vi "MGCC_StaEst_main_v2.vi"() -> ()   [LabVIEW 2016]
uses:
  <vilib>/imath/engines/lvmath2/RunTimeEngine/IndexRead/NIMS M(S,S).vi
  <instcachedir>/0/NIMS M(S,S)_AC51E74150A542F7991B9634C66F3096.lvgen/NIMS M(S,S)_AC51E74150A542F7991B9634C66F3096_001.vi
  <vilib>/imath/engines/lvmath2/RunTimeEngine/BuiltInFunctions/abs/NIMS_abs(signed).vi
  <instcachedir>/0/NIMS_abs(signed)_C4FCB8E6058B49B797C7C8D53CA5F6EC.lvgen/NIMS_abs(signed)_C4FCB8E6058B49B797C7C8D53CA5F6EC_002.vi
  <vilib>/imath/engines/lvmath2/RunTimeEngine/RunTimeType/NIMS_RunTimeType_From StrictType (excl LVString).vi
  <instcachedir>/0/NIMS_RunTimeType_From StrictType (excl LVString)_BBF44FB49F834B71AF7A14CCEDF8BECD.lvgen/NIMS_RunTimeType_From StrictType (excl LVString)_BBF44FB49F834B71AF7A14CCEDF8BECD_031.vi
  <vilib>/imath/engines/lvmath2/RunTimeEngine/Struct/NIMS_StructSetField.vi
  <vilib>/imathl/engines/lvmath/Functions/Error Handling/Create Error.vi
  <vilib>/imath/engines/lvmath2/RunTimeEngine/Struct/NIMS_StructGetField.vi
  <vilib>/imath/engines/lvmath2/RunTimeEngine/RunTimeType/NIMS_RunTimeType_To Numeric.vi
  <instcachedir>/0/NIMS_RunTimeType_To Numeric_19D51BCABB82435A94073491761E42EE.lvgen/NIMS_RunTimeType_To Numeric_19D51BCABB82435A94073491761E42EE_008.vi
  <instcachedir>/0/NIMS_RunTimeType_From StrictType (excl LVString)_BBF44FB49F834B71AF7A14CCEDF8BECD.lvgen/NIMS_RunTimeType_From StrictType (excl LVString)_BBF44FB49F834B71AF7A14CCEDF8BECD_000.vi
  <instcachedir>/0/NIMS_RunTimeType_To Numeric_19D51BCABB82435A94073491761E42EE.lvgen/NIMS_RunTimeType_To Numeric_19D51BCABB82435A94073491761E42EE_000.vi
  <vilib>/imath/engines/lvmath2/RunTimeEngine/IndexRead/NIMS M($,R2).vi
  <instcachedir>/0/NIMS M($,R2)_D9380E19261A4ADFB2D364AF6959C6EF.lvgen/NIMS M($,R2)_D9380E19261A4ADFB2D364AF6959C6EF_000.vi
  <instcachedir>/0/NIMS_RunTimeType_From StrictType (excl LVString)_BBF44FB49F834B71AF7A14CCEDF8BECD.lvgen/NIMS_RunTimeType_From StrictType (excl LVString)_BBF44FB49F834B71AF7A14CCEDF8BECD_009.vi
  <vilib>/imath/engines/lvmath2/RunTimeEngine/BuiltInFunctions/imag/NIMS_imag(Complex).vi
  <instcachedir>/0/NIMS_imag(Complex)_3180D40D00C843A49C2B33397F857BF3.lvgen/NIMS_imag(Complex)_3180D40D00C843A49C2B33397F857BF3_001.vi
  <instcachedir>/0/NIMS_abs(signed)_C4FCB8E6058B49B797C7C8D53CA5F6EC.lvgen/NIMS_abs(signed)_C4FCB8E6058B49B797C7C8D53CA5F6EC_003.vi
  <vilib>/imath/engines/lvmath2/RunTimeEngine/BuiltInFunctions/angle/NIMS_angle.vi
  <instcachedir>/0/NIMS_angle_6DDAE2BD99E0421EB990B6436E94D88F.lvgen/NIMS_angle_6DDAE2BD99E0421EB990B6436E94D88F_001.vi
  <instcachedir>/0/NIMS_RunTimeType_To Numeric_19D51BCABB82435A94073491761E42EE.lvgen/NIMS_RunTimeType_To Numeric_19D51BCABB82435A94073491761E42EE_003.vi
  <instcachedir>/0/NIMS_abs(signed)_C4FCB8E6058B49B797C7C8D53CA5F6EC.lvgen/NIMS_abs(signed)_C4FCB8E6058B49B797C7C8D53CA5F6EC_005.vi
  <vilib>/imath/engines/lvmath2/RunTimeEngine/VariableToken/Support/NIMS_Matrix Boolean Index to I32 Index.vi
  <vilib>/imath/engines/lvmath2/RunTimeEngine/IndexReplace/NIMS M(V)=S.vi
  <instcachedir>/0/NIMS M(V)=S_F2304187E1344F60ABCBE5C5CC0920F9.lvgen/NIMS M(V)=S_F2304187E1344F60ABCBE5C5CC0920F9_000.vi
  <instcachedir>/0/NIMS M($,R2)_D9380E19261A4ADFB2D364AF6959C6EF.lvgen/NIMS M($,R2)_D9380E19261A4ADFB2D364AF6959C6EF_001.vi
  <instcachedir>/0/NIMS_RunTimeType_From StrictType (excl LVString)_BBF44FB49F834B71AF7A14CCEDF8BECD.lvgen/NIMS_RunTimeType_From StrictType (excl LVString)_BBF44FB49F834B71AF7A14CCEDF8BECD_032.vi
  <instcachedir>/0/NIMS_RunTimeType_From StrictType (excl LVString)_BBF44FB49F834B71AF7A14CCEDF8BECD.lvgen/NIMS_RunTimeType_From StrictType (excl LVString)_BBF44FB49F834B71AF7A14CCEDF8BECD_024.vi
  LabVIEW Data/MathScriptVIs/MCStatic_36913154532_e94463401f82ecd62a182994faf25da2.vi
  <instcachedir>/0/MCStatic_36913154532_e94463401f82ecd62a182994faf25da2_D5C5374974BB412B8DCFE71036B3BD4D.lvgen/MCStatic_36913154532_e94463401f82ecd62a182994faf25da2_D5C5374974BB412B8DCFE71036B3BD4D_000.vi
  <instcachedir>/0/NIMS_RunTimeType_To Numeric_19D51BCABB82435A94073491761E42EE.lvgen/NIMS_RunTimeType_To Numeric_19D51BCABB82435A94073491761E42EE_009.vi
  <instcachedir>/0/NIMS_RunTimeType_To Numeric_19D51BCABB82435A94073491761E42EE.lvgen/NIMS_RunTimeType_To Numeric_19D51BCABB82435A94073491761E42EE_010.vi
  <vilib>/imath/engines/lvmath2/RunTimeEngine/BuiltInFunctions/size/NIMS_I32=size(GCol,I32).vi
  <instcachedir>/0/NIMS_I32=size(GCol,I32)_3BEAC9C04C22472CB193ADA08E7FE41C.lvgen/NIMS_I32=size(GCol,I32)_3BEAC9C04C22472CB193ADA08E7FE41C_000.vi
  <vilib>/imath/engines/lvmath2/RunTimeEngine/RangeToken/NIMS_Range_R2 - Integer.vi
  <instcachedir>/0/NIMS_Range_R2 - Integer_89B873E74E6E489885E44F751DD9C6BF.lvgen/NIMS_Range_R2 - Integer_89B873E74E6E489885E44F751DD9C6BF_000.vi
  <vilib>/imath/engines/lvmath2/RunTimeEngine/CommandStatement/MC_CommandStatement_break.vi
  <vilib>/imath/engines/lvmath2/RunTimeEngine/IndexRead/NIMS V(S).vi
  <instcachedir>/0/NIMS V(S)_0488751826AF41519A22953C041130DC.lvgen/NIMS V(S)_0488751826AF41519A22953C041130DC_002.vi
  <vilib>/imath/engines/lvmath2/RunTimeEngine/MatrixToken/NIMS_MatrixToken_M_RV.vi
  <instcachedir>/0/NIMS_MatrixToken_M_RV_EE14907D4B194E829889005D2F556E9C.lvgen/NIMS_MatrixToken_M_RV_EE14907D4B194E829889005D2F556E9C_002.vi
  <vilib>/imath/engines/lvmath2/RunTimeEngine/ErrorHandling/NIMS_Create Error From Enums.vi
  LabVIEW Data/MathScriptVIs/MCStatic_36913154532_cdc492c47a81eb15c08497af6b311993.vi
  <instcachedir>/0/MCStatic_36913154532_cdc492c47a81eb15c08497af6b311993_54503743F61444378DD671EE6F584E70.lvgen/MCStatic_36913154532_cdc492c47a81eb15c08497af6b311993_54503743F61444378DD671EE6F584E70_000.vi
  <vilib>/imath/engines/lvmath2/RunTimeEngine/RangeToken/NIMS_Range.vi
  <instcachedir>/0/NIMS_Range_A7C094595B484CA7AF10685B02D808ED.lvgen/NIMS_Range_A7C094595B484CA7AF10685B02D808ED_000.vi
  <vilib>/imath/engines/lvmath2/RunTimeEngine/MatrixToken/NIMS_MatrixToken_M_SorCV.vi
  <instcachedir>/0/NIMS_MatrixToken_M_SorCV_D3266533510A4291A747E91CF193467A.lvgen/NIMS_MatrixToken_M_SorCV_D3266533510A4291A747E91CF193467A_000.vi
  LabVIEW Data/MathScriptVIs/MCStatic_36913154532_c8cdcb96f1d039e13ab6944736b2cbcd.vi
  <instcachedir>/0/MCStatic_36913154532_c8cdcb96f1d039e13ab6944736b2cbcd_6DF1093E75004D0A86BBD1CDE7CCB5DF.lvgen/MCStatic_36913154532_c8cdcb96f1d039e13ab6944736b2cbcd_6DF1093E75004D0A86BBD1CDE7CCB5DF_002.vi
  <vilib>/imath/engines/lvmath2/RunTimeEngine/BuiltInFunctions/rand/NIMS_rand(I32,I32).vi
  <vilib>/imath/engines/lvmath2/RunTimeEngine/ArithmeticOperatorToken/NIMS_ArithmeticOperator_plus.vi
  <instcachedir>/0/NIMS_ArithmeticOperator_plus_0120E0498A0F4B4B9BDCAC2554767A4E.lvgen/NIMS_ArithmeticOperator_plus_0120E0498A0F4B4B9BDCAC2554767A4E_009.vi
  <vilib>/imath/engines/lvmath2/RunTimeEngine/ErrorHandling/NIMS_Error From Error Code.vi
  <vilib>/imath/engines/lvmath/Functions/Error Handling/MergeErrorsWrapper.vi
  <vilib>/imath/engines/lvmath2/RunTimeEngine/ArithmeticOperatorToken/NIMS_ArithmeticOperator_times.vi
  <instcachedir>/0/NIMS_ArithmeticOperator_times_953B34F74CAC448FB707D816A29CC5F0.lvgen/NIMS_ArithmeticOperator_times_953B34F74CAC448FB707D816A29CC5F0_007.vi
  <vilib>/imath/engines/lvmath2/RunTimeEngine/BuiltInFunctions/reshapemx/NIMS_[GV]_reshapemx.vi
  <instcachedir>/0/NIMS_[GV]_reshapemx_314E456D64644EB191D4916921E89AA6.lvgen/NIMS_[GV]_reshapemx_314E456D64644EB191D4916921E89AA6_000.vi
  <vilib>/imath/engines/lvmath2/RunTimeSupport/NIMS_Error if Not Equal.vi
  <instcachedir>/0/NIMS_Error if Not Equal_43252A79AD05436189442EC0C5E5AB8A.lvgen/NIMS_Error if Not Equal_43252A79AD05436189442EC0C5E5AB8A_002.vi
  <vilib>/imath/engines/lvmath2/RunTimeEngine/IndexRead/NIMS M(M).vi
  <instcachedir>/0/NIMS M(M)_EB00EBD471DD47B0915ED9997EB5A993.lvgen/NIMS M(M)_EB00EBD471DD47B0915ED9997EB5A993_004.vi
  <vilib>/imath/engines/lvmath2/RunTimeEngine/MatrixToken/NIMS_MatrixToken_M_M.vi
  <instcachedir>/0/NIMS_MatrixToken_M_M_DF273B0CC20F424BBF1EDA9F4E71C841.lvgen/NIMS_MatrixToken_M_M_DF273B0CC20F424BBF1EDA9F4E71C841_004.vi
  <vilib>/imath/engines/lvmath2/RunTimeEngine/IndexRead/NIMS M($,S).vi
  <instcachedir>/0/NIMS M($,S)_3E5749BBB62E49528D4765A77F1F6D98.lvgen/NIMS M($,S)_3E5749BBB62E49528D4765A77F1F6D98_000.vi
  <vilib>/imath/engines/lvmath2/RunTimeEngine/BuiltInFunctions/size/NIMS_I32Row=size(GM).vi
  <instcachedir>/0/NIMS_I32Row=size(GM)_10ACDCB9F1F84A7E9F42C91D87611FB5.lvgen/NIMS_I32Row=size(GM)_10ACDCB9F1F84A7E9F42C91D87611FB5_001.vi
  <vilib>/imath/engines/lvmath2/RunTimeEngine/BuiltInFunctions/ones/NIMS_M=ones(I32V).vi
  <vilib>/imath/engines/lvmath2/RunTimeEngine/BuiltInFunctions/diag/NIMS_diag.vi
  <instcachedir>/0/NIMS_diag_BAFF033CE85645D0951408836EA255EA.lvgen/NIMS_diag_BAFF033CE85645D0951408836EA255EA_003.vi
  <vilib>/imath/engines/lvmath2/RunTimeEngine/RowToken/NIMS_RowToken_CV_CV.vi
  <instcachedir>/0/NIMS_RowToken_CV_CV_5546A0B1CA2C4E49826F811B9C073FB0.lvgen/NIMS_RowToken_CV_CV_5546A0B1CA2C4E49826F811B9C073FB0_000.vi
  <vilib>/imath/engines/lvmath2/RunTimeEngine/BuiltInFunctions/zeros/NIMS_M=zeros(I32,I32).vi
  <vilib>/imath/engines/lvmath2/RunTimeEngine/RangeToken/NIMS_Range_R2 - Float.vi
  <instcachedir>/0/NIMS_Range_R2 - Float_590A1087448447AEB7F770FC082D3801.lvgen/NIMS_Range_R2 - Float_590A1087448447AEB7F770FC082D3801_000.vi
  <instcachedir>/0/NIMS_Error if Not Equal_43252A79AD05436189442EC0C5E5AB8A.lvgen/NIMS_Error if Not Equal_43252A79AD05436189442EC0C5E5AB8A_000.vi
  <instcachedir>/0/NIMS M(S,S)_AC51E74150A542F7991B9634C66F3096.lvgen/NIMS M(S,S)_AC51E74150A542F7991B9634C66F3096_000.vi
  <vilib>/imath/engines/lvmath2/RunTimeEngine/IndexReplace/NIMS M(S,S)=S.vi
  <instcachedir>/0/NIMS M(S,S)=S_98E40400474E4398B113AE20298B4F82.lvgen/NIMS M(S,S)=S_98E40400474E4398B113AE20298B4F82_000.vi
  LabVIEW Data/MathScriptVIs/MCStatic_36913154532_d43c7c68f2dc95cb57c489aed42a4476.vi
  <instcachedir>/0/MCStatic_36913154532_d43c7c68f2dc95cb57c489aed42a4476_C67C1925C8044DA9AFBC9BF5A01EA825.lvgen/MCStatic_36913154532_d43c7c68f2dc95cb57c489aed42a4476_C67C1925C8044DA9AFBC9BF5A01EA825_000.vi
  LabVIEW Data/MathScriptVIs/MCStatic_36913154532_67c6299701e115b47b312b72959cc131.vi
  <instcachedir>/0/MCStatic_36913154532_67c6299701e115b47b312b72959cc131_A8DF1F8A1F0E4CF3AEF72F0B4F2CA190.lvgen/MCStatic_36913154532_67c6299701e115b47b312b72959cc131_A8DF1F8A1F0E4CF3AEF72F0B4F2CA190_000.vi
  <vilib>/imath/engines/lvmath2/RunTimeEngine/IndexReplace/NIMS M($,V)=S.vi
  <instcachedir>/0/NIMS M($,V)=S_8FF4B0FF94A24B3598424F2A899DBD06.lvgen/NIMS M($,V)=S_8FF4B0FF94A24B3598424F2A899DBD06_000.vi
  <instcachedir>/0/NIMS_Error if Not Equal_43252A79AD05436189442EC0C5E5AB8A.lvgen/NIMS_Error if Not Equal_43252A79AD05436189442EC0C5E5AB8A_001.vi
  LabVIEW Data/MathScriptVIs/MCStatic_36913154532_0e35dc52ff3fcf820f0ec3822af42f61.vi
  <instcachedir>/0/MCStatic_36913154532_0e35dc52ff3fcf820f0ec3822af42f61_1384647D6A3B401EB7EF92DE69A0FCD8.lvgen/MCStatic_36913154532_0e35dc52ff3fcf820f0ec3822af42f61_1384647D6A3B401EB7EF92DE69A0FCD8_000.vi
  LabVIEW Data/MathScriptVIs/MCStatic_36913154532_31a3e73c3b07f43dd7c3efcbba35961a.vi
  <instcachedir>/0/MCStatic_36913154532_31a3e73c3b07f43dd7c3efcbba35961a_F912710ABE814275AC6B55EC75CD9760.lvgen/MCStatic_36913154532_31a3e73c3b07f43dd7c3efcbba35961a_F912710ABE814275AC6B55EC75CD9760_000.vi
  <vilib>/imath/engines/lvmath2/RunTimeEngine/ArithmeticOperatorToken/NIMS_ArithmeticOperator_minus.vi
  <instcachedir>/0/NIMS_ArithmeticOperator_minus_E3B65B1D26A44BB184AFDC5B3F458E3D.lvgen/NIMS_ArithmeticOperator_minus_E3B65B1D26A44BB184AFDC5B3F458E3D_003.vi
  <vilib>/imath/engines/lvmath2/RunTimeEngine/ArithmeticOperatorToken/NIMS_ArithmeticOperator_rightdivmx.vi
  <instcachedir>/0/NIMS_ArithmeticOperator_rightdivmx_0DBBD6F2821B4AB59571CD9AB2DE9D62.lvgen/NIMS_ArithmeticOperator_rightdivmx_0DBBD6F2821B4AB59571CD9AB2DE9D62_000.vi
  <vilib>/imath/engines/lvmath2/RunTimeEngine/ArithmeticOperatorToken/NIMS_ArithmeticOperator_multmx(M,CV).vi
  <instcachedir>/0/NIMS_ArithmeticOperator_multmx(M,CV)_EE734FC8520844C9A7CC1A67008668A3.lvgen/NIMS_ArithmeticOperator_multmx(M,CV)_EE734FC8520844C9A7CC1A67008668A3_000.vi
  <vilib>/imath/engines/lvmath2/RunTimeEngine/ArithmeticOperatorToken/NIMS_ArithmeticOperator_multmx.vi
  <instcachedir>/0/NIMS_ArithmeticOperator_multmx_4A56FE5C615140CE835D4DB5891BF065.lvgen/NIMS_ArithmeticOperator_multmx_4A56FE5C615140CE835D4DB5891BF065_004.vi
  <vilib>/imath/engines/lvmath2/RunTimeEngine/BuiltInFunctions/pinv/NIMS_pinv.vi
  <instcachedir>/0/NIMS_pinv_206F0700CF75499C820074BA4F1FFC36.lvgen/NIMS_pinv_206F0700CF75499C820074BA4F1FFC36_000.vi
  LabVIEW Data/MathScriptVIs/MCStatic_36913154532_3e0713edee310e467a0af9b75de98b5e.vi
  <instcachedir>/0/MCStatic_36913154532_3e0713edee310e467a0af9b75de98b5e_43634E09506847119E5765429ED34CE7.lvgen/MCStatic_36913154532_3e0713edee310e467a0af9b75de98b5e_43634E09506847119E5765429ED34CE7_000.vi
  LabVIEW Data/MathScriptVIs/MCStatic_36913154532_2702dd0801db0973dda6904d586f103d.vi
  <instcachedir>/0/MCStatic_36913154532_2702dd0801db0973dda6904d586f103d_BD9A4538893B490BA7661E5823328DB1.lvgen/MCStatic_36913154532_2702dd0801db0973dda6904d586f103d_BD9A4538893B490BA7661E5823328DB1_000.vi
  <instcachedir>/0/NIMS_ArithmeticOperator_minus_E3B65B1D26A44BB184AFDC5B3F458E3D.lvgen/NIMS_ArithmeticOperator_minus_E3B65B1D26A44BB184AFDC5B3F458E3D_002.vi
  <vilib>/imath/engines/lvmath2/RunTimeEngine/BuiltInFunctions/max/1 input/NIMS_max(RM).vi
  <instcachedir>/0/NIMS_max(RM)_358AE92FF7FA4D91BF0D9DEC69043403.lvgen/NIMS_max(RM)_358AE92FF7FA4D91BF0D9DEC69043403_000.vi
  <instcachedir>/0/NIMS_ArithmeticOperator_plus_0120E0498A0F4B4B9BDCAC2554767A4E.lvgen/NIMS_ArithmeticOperator_plus_0120E0498A0F4B4B9BDCAC2554767A4E_003.vi
  <vilib>/imath/engines/lvmath2/RunTimeEngine/VariableToken/NIMS_VariableToken_CondDefined.vi
  <instcachedir>/0/NIMS_VariableToken_CondDefined_06E9DA95BD4D46A6BA55EC651A891960.lvgen/NIMS_VariableToken_CondDefined_06E9DA95BD4D46A6BA55EC651A891960_001.vi
  <instcachedir>/0/NIMS_VariableToken_CondDefined_06E9DA95BD4D46A6BA55EC651A891960.lvgen/NIMS_VariableToken_CondDefined_06E9DA95BD4D46A6BA55EC651A891960_005.vi
  <vilib>/imath/engines/lvmath2/RunTimeEngine/IndexRead/NIMS M(V).vi
  <instcachedir>/0/NIMS M(V)_948FAC22C1C943948B75DA6190348614.lvgen/NIMS M(V)_948FAC22C1C943948B75DA6190348614_005.vi
  <vilib>/imath/engines/lvmath2/RunTimeEngine/BuiltInFunctions/reshapemx/NIMS_[GM]_reshapemx.vi
  <instcachedir>/0/NIMS_[GM]_reshapemx_500BD31B48F5434EA23B2056DCB44201.lvgen/NIMS_[GM]_reshapemx_500BD31B48F5434EA23B2056DCB44201_000.vi
  <instcachedir>/0/NIMS_ArithmeticOperator_plus_0120E0498A0F4B4B9BDCAC2554767A4E.lvgen/NIMS_ArithmeticOperator_plus_0120E0498A0F4B4B9BDCAC2554767A4E_010.vi
  <instcachedir>/0/NIMS_VariableToken_CondDefined_06E9DA95BD4D46A6BA55EC651A891960.lvgen/NIMS_VariableToken_CondDefined_06E9DA95BD4D46A6BA55EC651A891960_006.vi
  <instcachedir>/0/NIMS_VariableToken_CondDefined_06E9DA95BD4D46A6BA55EC651A891960.lvgen/NIMS_VariableToken_CondDefined_06E9DA95BD4D46A6BA55EC651A891960_003.vi
  <vilib>/imath/engines/lvmath2/RunTimeEngine/NodeEndStatement/NIMS_NodeEndStatement_Output.vi
  <instcachedir>/0/NIMS_NodeEndStatement_Output_53EC0D466D134D7ABD903AC30B43404B.lvgen/NIMS_NodeEndStatement_Output_53EC0D466D134D7ABD903AC30B43404B_011.vi
  <instcachedir>/0/NIMS_NodeEndStatement_Output_53EC0D466D134D7ABD903AC30B43404B.lvgen/NIMS_NodeEndStatement_Output_53EC0D466D134D7ABD903AC30B43404B_005.vi
  <instcachedir>/0/NIMS_NodeEndStatement_Output_53EC0D466D134D7ABD903AC30B43404B.lvgen/NIMS_NodeEndStatement_Output_53EC0D466D134D7ABD903AC30B43404B_002.vi
  <instcachedir>/0/NIMS_NodeEndStatement_Output_53EC0D466D134D7ABD903AC30B43404B.lvgen/NIMS_NodeEndStatement_Output_53EC0D466D134D7ABD903AC30B43404B_003.vi
  <instcachedir>/0/NIMS_NodeEndStatement_Output_53EC0D466D134D7ABD903AC30B43404B.lvgen/NIMS_NodeEndStatement_Output_53EC0D466D134D7ABD903AC30B43404B_001.vi
  <instcachedir>/0/NIMS_NodeEndStatement_Output_53EC0D466D134D7ABD903AC30B43404B.lvgen/NIMS_NodeEndStatement_Output_53EC0D466D134D7ABD903AC30B43404B_024.vi
  <instcachedir>/0/NIMS_NodeEndStatement_Output_53EC0D466D134D7ABD903AC30B43404B.lvgen/NIMS_NodeEndStatement_Output_53EC0D466D134D7ABD903AC30B43404B_015.vi
  <instcachedir>/0/NIMS_NodeEndStatement_Output_53EC0D466D134D7ABD903AC30B43404B.lvgen/NIMS_NodeEndStatement_Output_53EC0D466D134D7ABD903AC30B43404B_013.vi
  <instcachedir>/0/NIMS_NodeEndStatement_Output_53EC0D466D134D7ABD903AC30B43404B.lvgen/NIMS_NodeEndStatement_Output_53EC0D466D134D7ABD903AC30B43404B_021.vi
  <instcachedir>/0/NIMS_NodeEndStatement_Output_53EC0D466D134D7ABD903AC30B43404B.lvgen/NIMS_NodeEndStatement_Output_53EC0D466D134D7ABD903AC30B43404B_018.vi
  <instcachedir>/0/NIMS_NodeEndStatement_Output_53EC0D466D134D7ABD903AC30B43404B.lvgen/NIMS_NodeEndStatement_Output_53EC0D466D134D7ABD903AC30B43404B_022.vi
  <instcachedir>/0/NIMS_NodeEndStatement_Output_53EC0D466D134D7ABD903AC30B43404B.lvgen/NIMS_NodeEndStatement_Output_53EC0D466D134D7ABD903AC30B43404B_020.vi
  <instcachedir>/0/NIMS_NodeEndStatement_Output_53EC0D466D134D7ABD903AC30B43404B.lvgen/NIMS_NodeEndStatement_Output_53EC0D466D134D7ABD903AC30B43404B_028.vi
  <instcachedir>/0/NIMS_NodeEndStatement_Output_53EC0D466D134D7ABD903AC30B43404B.lvgen/NIMS_NodeEndStatement_Output_53EC0D466D134D7ABD903AC30B43404B_004.vi
  <instcachedir>/0/NIMS_NodeEndStatement_Output_53EC0D466D134D7ABD903AC30B43404B.lvgen/NIMS_NodeEndStatement_Output_53EC0D466D134D7ABD903AC30B43404B_014.vi
  <instcachedir>/0/NIMS_NodeEndStatement_Output_53EC0D466D134D7ABD903AC30B43404B.lvgen/NIMS_NodeEndStatement_Output_53EC0D466D134D7ABD903AC30B43404B_027.vi
  <vilib>/imath/engines/lvmath2/RunTimeEngine/ErrorHandling/NIMS_Finalize Error.vi
  Sub-VIs/idx2pha.m
  Sub-VIs/pha2idx.m
  Sub-VIs/zeroinjec.m
  Sub-VIs/cequ.m
  Sub-VIs/cjoc.m
  Sub-VIs/pnequ.m
  Sub-VIs/pnjoc.m
  Sub-VIs/vnequ.m
  Sub-VIs/vnjoc.m
  <instcachedir>/0/MCStatic_36913154532_0e35dc52ff3fcf820f0ec3822af42f61_1384647D6A3B401EB7EF92DE69A0FCD8.lvgen/MCStatic_36913154532_0e35dc52ff3fcf820f0ec3822af42f61_1384647D6A3B401EB7EF92DE69A0FCD8_001.vi
  <instcachedir>/0/MCStatic_36913154532_2702dd0801db0973dda6904d586f103d_BD9A4538893B490BA7661E5823328DB1.lvgen/MCStatic_36913154532_2702dd0801db0973dda6904d586f103d_BD9A4538893B490BA7661E5823328DB1_001.vi
  <instcachedir>/0/MCStatic_36913154532_31a3e73c3b07f43dd7c3efcbba35961a_F912710ABE814275AC6B55EC75CD9760.lvgen/MCStatic_36913154532_31a3e73c3b07f43dd7c3efcbba35961a_F912710ABE814275AC6B55EC75CD9760_001.vi
  <instcachedir>/0/MCStatic_36913154532_67c6299701e115b47b312b72959cc131_A8DF1F8A1F0E4CF3AEF72F0B4F2CA190.lvgen/MCStatic_36913154532_67c6299701e115b47b312b72959cc131_A8DF1F8A1F0E4CF3AEF72F0B4F2CA190_001.vi
  <instcachedir>/0/MCStatic_36913154532_d43c7c68f2dc95cb57c489aed42a4476_C67C1925C8044DA9AFBC9BF5A01EA825.lvgen/MCStatic_36913154532_d43c7c68f2dc95cb57c489aed42a4476_C67C1925C8044DA9AFBC9BF5A01EA825_001.vi
panel:
  out "index":i32
  out "puTrue":T1
  out "Num":T2
  out "Loc":cluster{"Zeroinj":i32[][], "Line":dbl[][]}
  out "seResult":T3
  out "str_MGCC_MdlMgmt_Feeder":T4
  out "error out":errorcluster
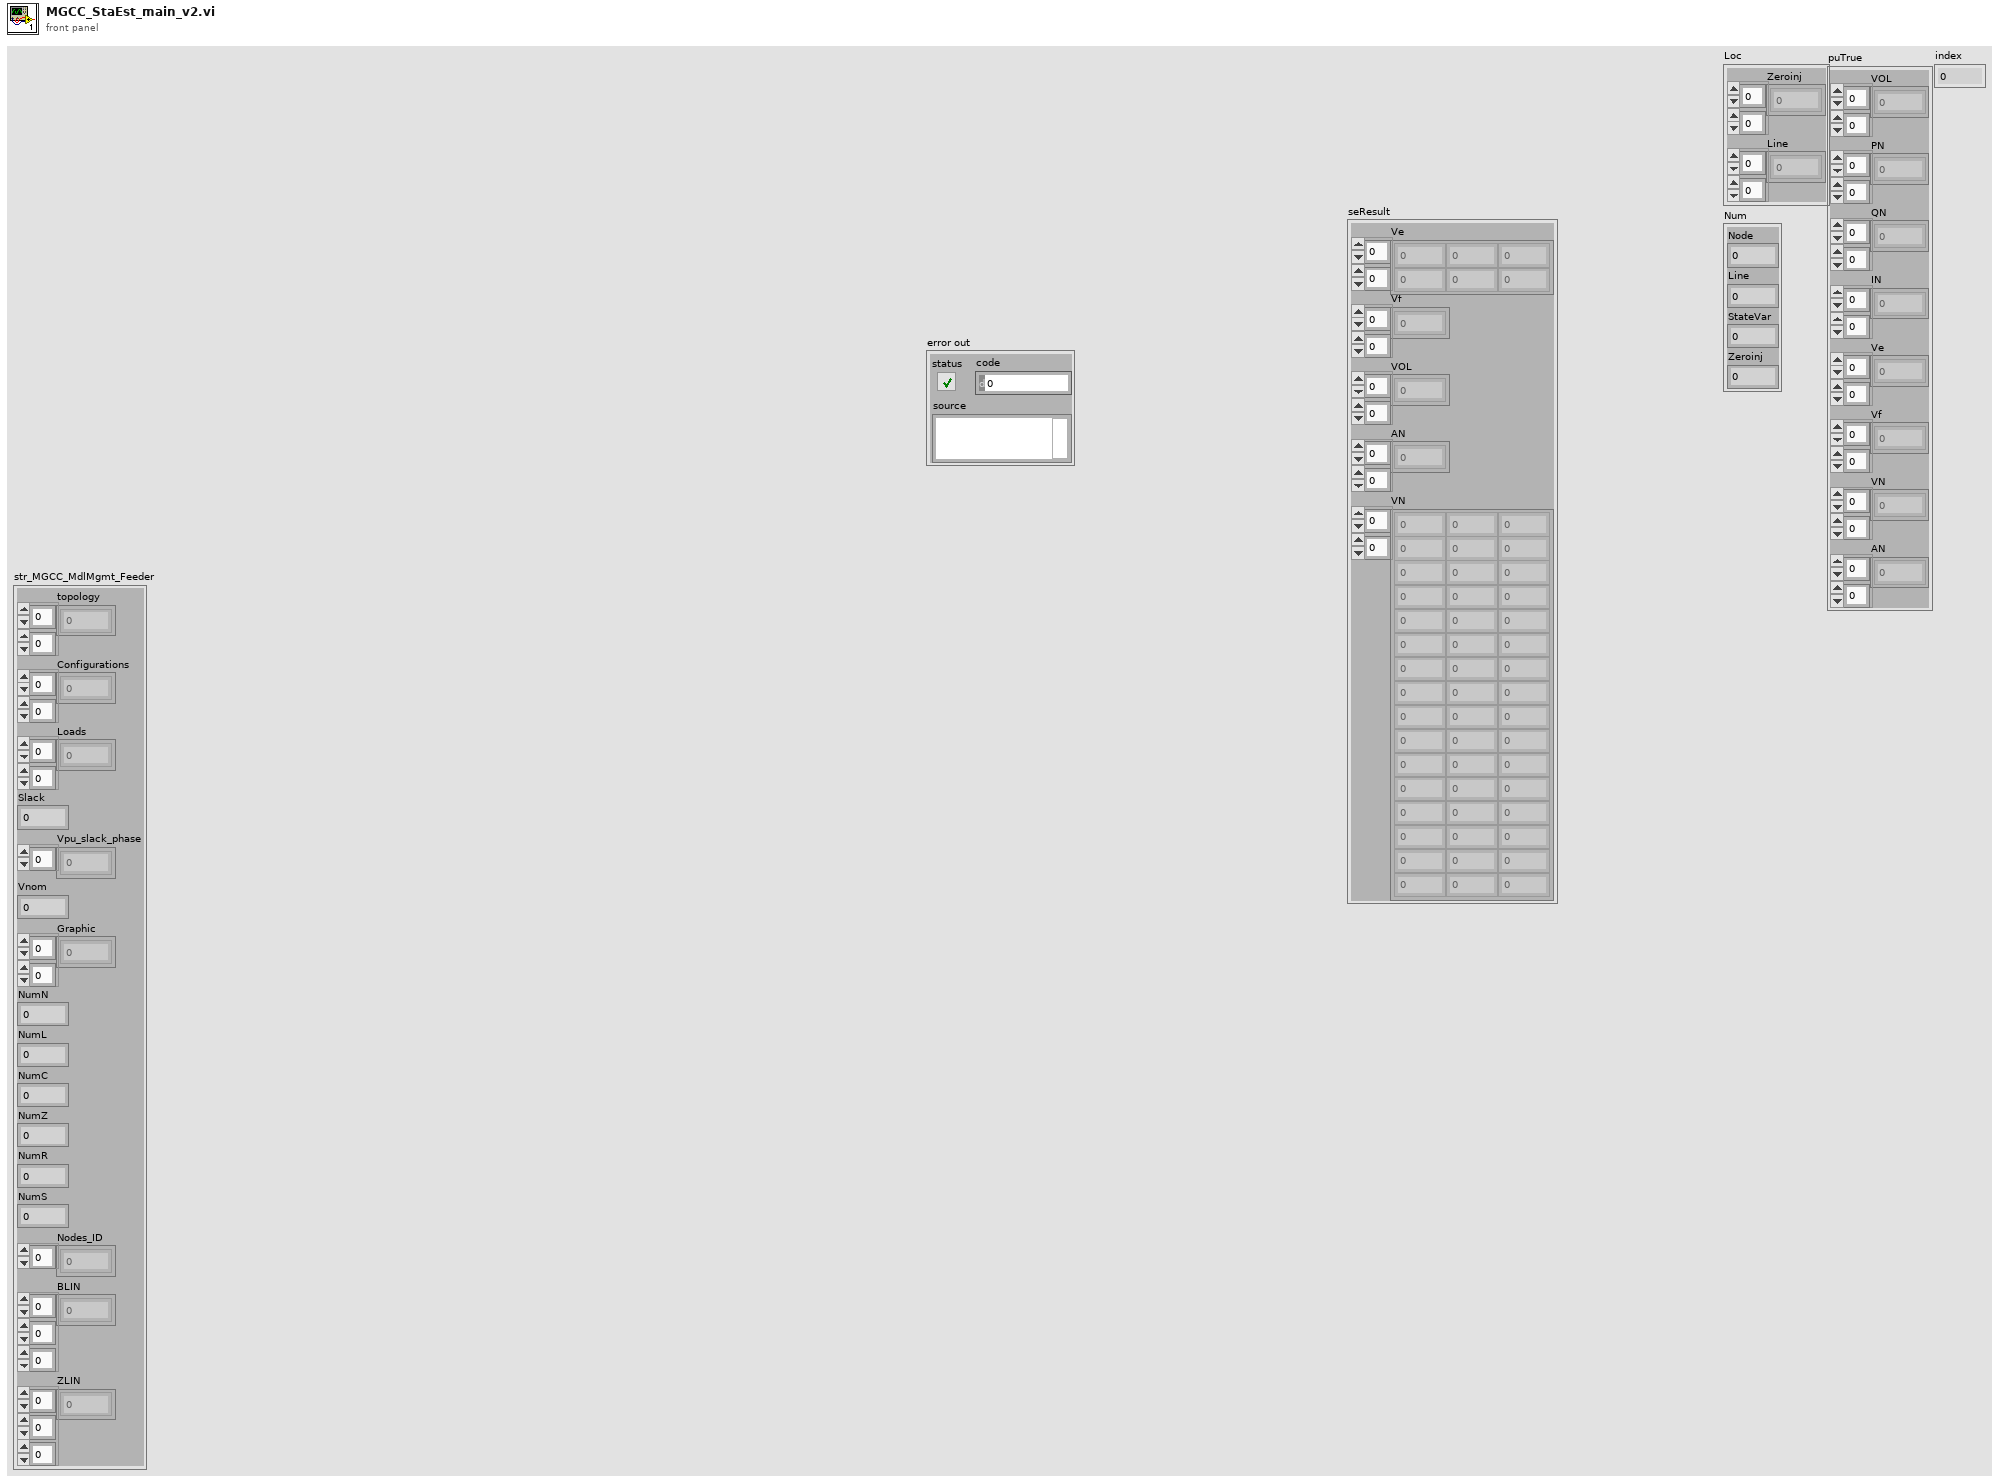
[diagram p1: front panel]
types:
  T1 = cluster{"VOL":cdb[][], "PN":dbl[][], "QN":dbl[][], "IN":dbl[][], "Ve":dbl[][], "Vf":dbl[][], "VN":dbl[][], "AN":dbl[][]}
  T2 = cluster{"Node":dbl, "Line":dbl, "StateVar":i32, "Zeroinj":i32}
  T3 = cluster{"Ve":dbl[][], "Vf":dbl[][], "VOL":cdb[][], "AN":dbl[][], "VN":dbl[][]}
  T4 = cluster{"topology":dbl[][], "Configurations":dbl[][], "Loads":dbl[][], "Slack":dbl, "Vpu_slack_phase":cdb[], "Vnom":dbl, "Graphic":dbl[][], "NumN":dbl, "NumL":dbl, "NumC":dbl, "NumZ":dbl, "NumR":dbl, "NumS":dbl, "Nodes_ID":dbl[], "BLIN":cdb[][][], "ZLIN":cdb[][][]}
  T5 = cluster{"PN":dbl[][], "QN":dbl[][], "VN":dbl[][]}
  T6 = cluster{"Sbase":dbl, "Vbase":dbl, "Ibase":dbl, "Ybase":dbl}
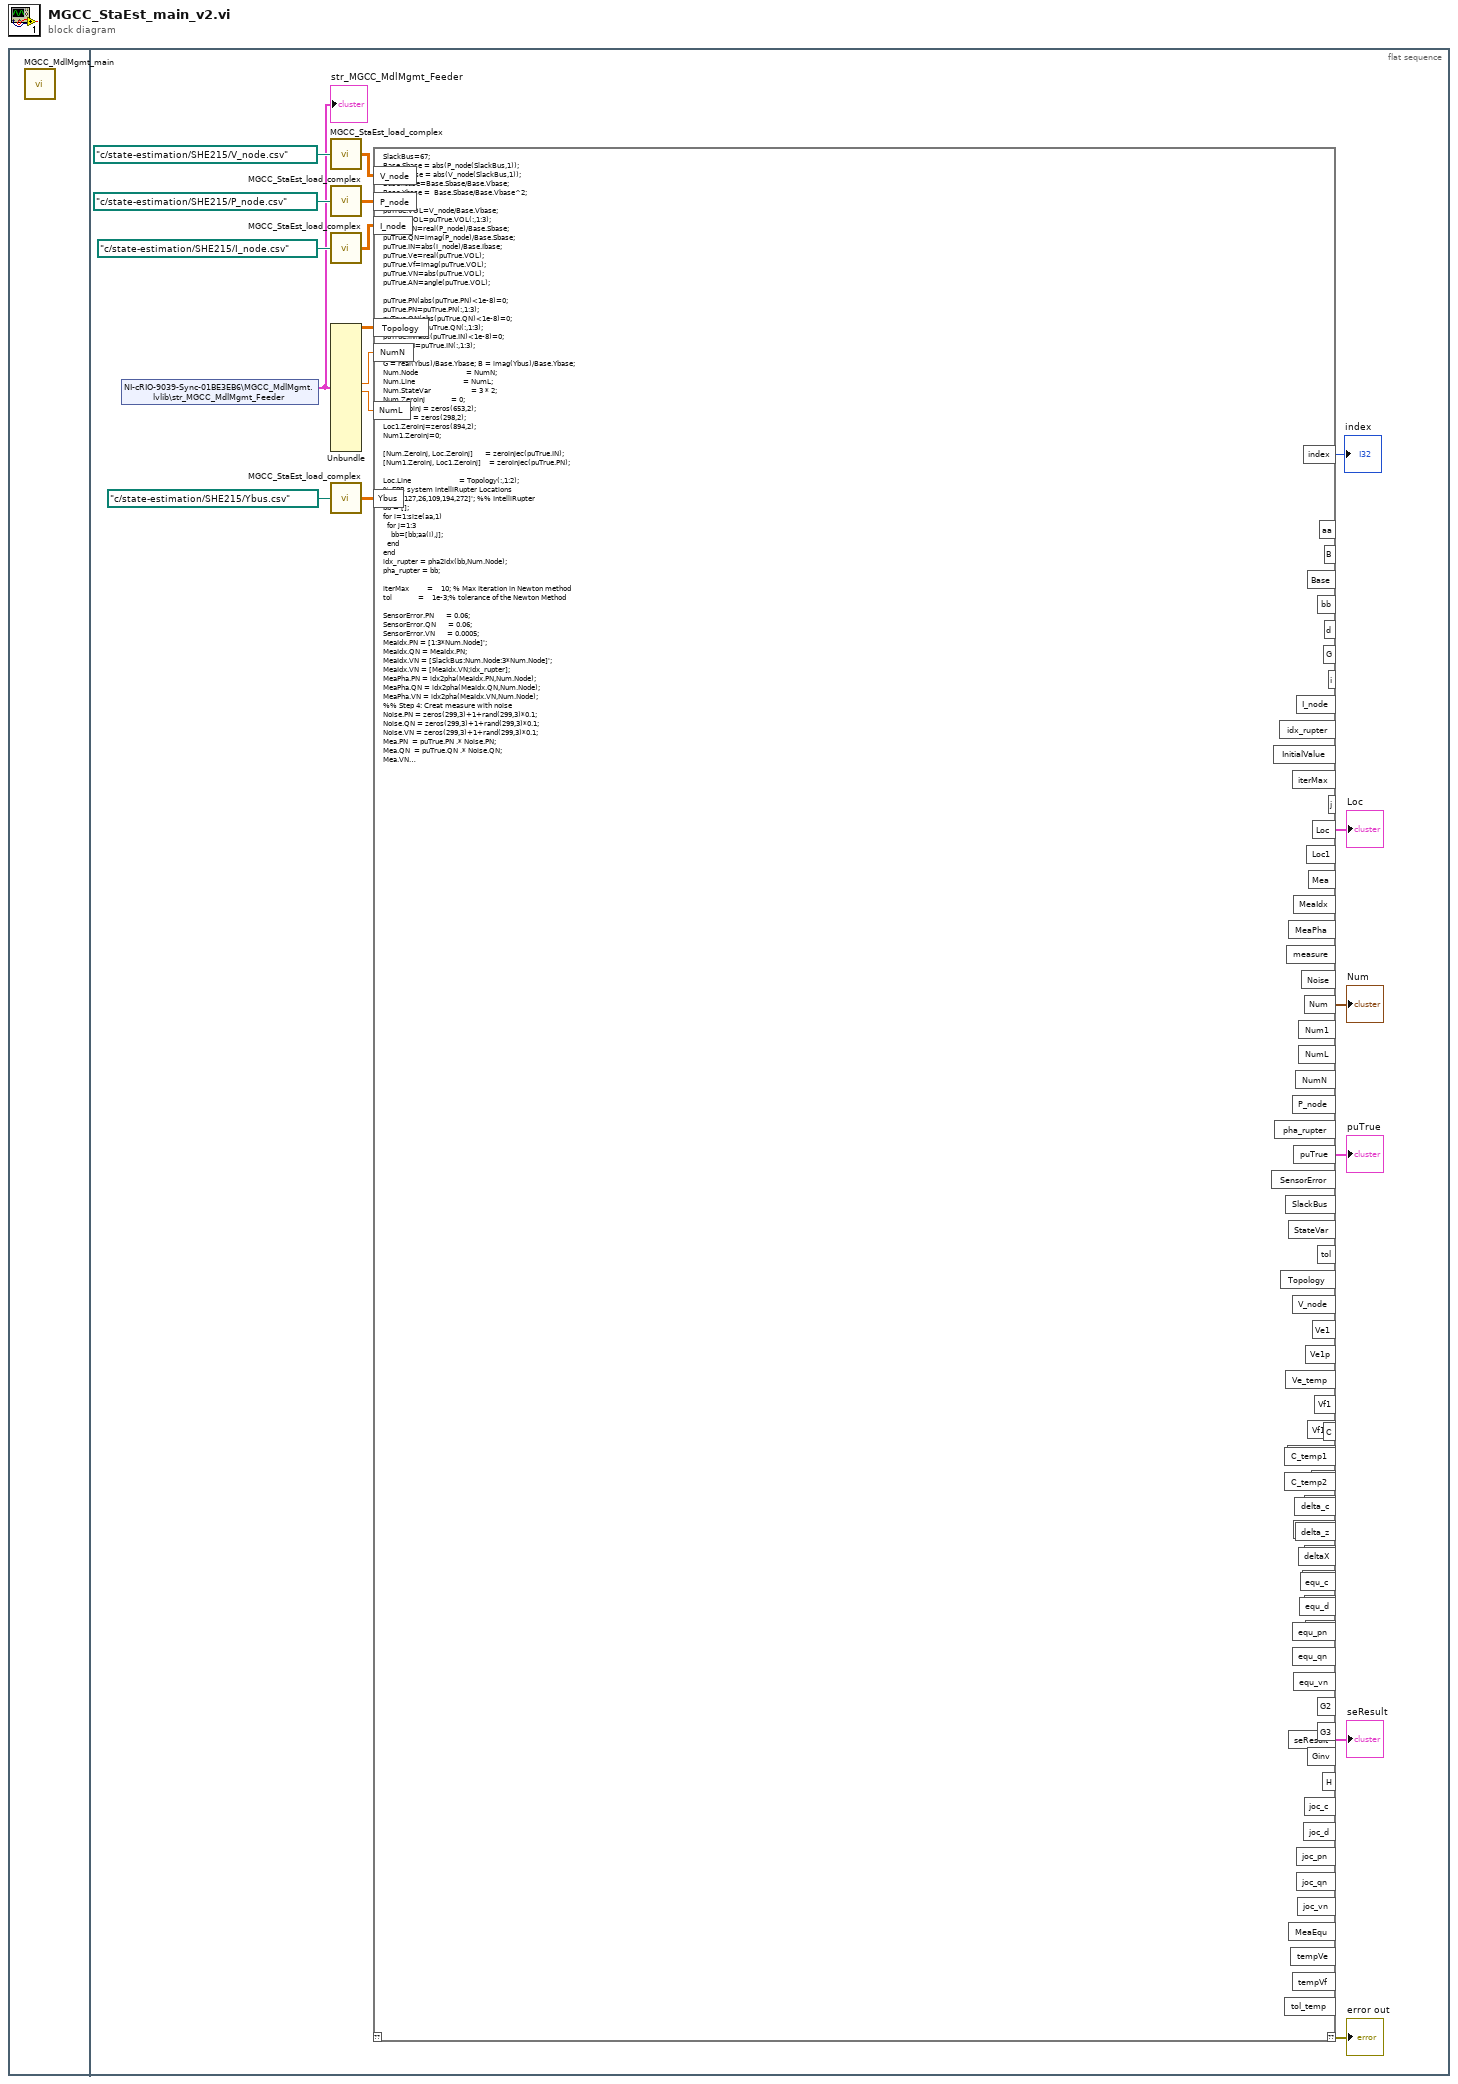
[diagram p0: block diagram]
diagram:
  n1 = flat-sequence {
    frame #0 {
      n2 = call "MGCC_MdlMgmt_main.vi"() -> ()  [unwired: 12 in]
    }
    frame #1 {
      n3 = shared-variable "NI-cRIO-9039-Sync-01BE3EB6\\MGCC_MdlMgmt.lvlib\\str_MGCC_MdlMgmt_Feeder"() -> (w11:T4)  [unwired: 1 in, 1 out]
      "str_MGCC_MdlMgmt_Feeder" <- w11
      n4 = call "MGCC_StaEst_load_complex.vi"("file path (dialog if empty)"=path "c:/state-estimation/SHE215/V_node.csv" ("file path (use dialog)")) -> ("Array 13"=w14:cdb[][])
      n5 = call "MGCC_StaEst_load_complex.vi"("file path (dialog if empty)"=path "c:/state-estimation/SHE215/P_node.csv" ("file path (use dialog)")) -> ("Array 13"=w13:cdb[][])
      n6 = call "MGCC_StaEst_load_complex.vi"("file path (dialog if empty)"=path "c:/state-estimation/SHE215/I_node.csv" ("file path (use dialog)")) -> ("Array 13"=w12:cdb[][])
      n7 = Unbundle(w11) -> ("topology"=w6:dbl[][], "NumN"=w10:dbl, "NumL"=w9:dbl)  [unwired: 13 out]
      n8 = call "MGCC_StaEst_load_complex.vi"("file path (dialog if empty)"=path "c:/state-estimation/SHE215/Ybus.csv" ("file path (use dialog)")) -> ("Array 13"=w7:cdb[][])
      n9 = mathscript code="SlackBus=67;\nBase.Sbase = abs(P_node(SlackBus,1));\nBase.Vbase = abs(V_node(SlackBus,1));\nBase.Ibase=Base.Sbase/Base.Vbase;\nBase.Ybase =  Base.Sbase/Base.Vbase^2;\n\npuTrue.VOL=V_node/Base.Vbase;\npuTrue.VOL=puTrue.VOL(:,1:3);\npuTrue.PN=real(P_node)/Base.Sbase;\npuTrue.QN=imag(P_node)/Base.Sbase;\npuTrue.IN=abs(I_node)/Base.Ibase;\npuTrue.Ve=real(puTrue.VOL);\npuTrue.Vf=imag(puTrue.VOL); \npuTrue.VN=abs(puTrue.VOL);\npuTrue.AN=angle(puTrue.VOL);\n\npuTrue.PN(abs(puTrue.PN)<1e-8)=0;\npuTrue.PN=puTrue.PN(:,1:3);\npuTrue.QN(abs(puTrue.QN)<1e-8)=0;\npuTrue.QN=puTrue.QN(:,1:3);\npuTrue.IN(abs(puTrue.IN)<1e-8)=0;\npuTrue.IN=puTrue.IN(:,1:3);\n\nG = real(Ybus)/Base.Ybase; B = imag(Ybus)/Base.Ybase;\nNum.Node                        = NumN;\nNum.Line                        = NumL;\nNum.StateVar                    = 3 * 2;  \nNum.Zeroinj             = 0;\nLoc.Zeroinj = zeros(653,2);\nLoc.Line = zeros(298,2);\nLoc1.Zeroinj=zeros(894,2);\nNum1.Zeroinj=0;\n\n[Num.Zeroinj, Loc.Zeroinj]      = zeroinjec(puTrue.IN);\n[Num1.Zeroinj, Loc1.Zeroinj]    = zeroinjec(puTrue.PN);\n\nLoc.Line                        = Topology(:,1:2);\n% EPB system intelliRupter Locations\naa = [127,26,109,194,272]'; %% IntelliRupter\nbb = [];\nfor i=1:size(aa,1)\n  for j=1:3\n    bb=[bb;aa(i),j];\n  end\nend\nidx_rupter = pha2idx(bb,Num.Node);\npha_rupter = bb;\n\niterMax         =    10; % Max Iteration in Newton method\ntol             =    1e-3;% tolerance of the Newton Method\n\nSensorError.PN      = 0.06;\nSensorError.QN      = 0.06;\nSensorError.VN      = 0.0005;\nMeaIdx.PN = [1:3*Num.Node]';\nMeaIdx.QN = MeaIdx.PN;\nMeaIdx.VN = [SlackBus:Num.Node:3*Num.Node]';\nMeaIdx.VN = [MeaIdx.VN;idx_rupter]; \nMeaPha.PN = idx2pha(MeaIdx.PN,Num.Node);\nMeaPha.QN = idx2pha(MeaIdx.QN,Num.Node);\nMeaPha.VN = idx2pha(MeaIdx.VN,Num.Node);\n%% Step 4: Creat measure with noise\nNoise.PN = zeros(299,3)+1+rand(299,3)*0.1;\nNoise.QN = zeros(299,3)+1+rand(299,3)*0.1;\nNoise.VN = zeros(299,3)+1+rand(299,3)*0.1;\nMea.PN  = puTrue.PN .* Noise.PN; \nMea.QN  = puTrue.QN .* Noise.QN;\nMea.VN  = puTrue.VN.^2 .* Noise.VN;\nMea.PN  = reshape(Mea.PN,3*Num.Node,1);\nMea.QN  = reshape(Mea.QN,3*Num.Node,1);\nMea.VN  = reshape(Mea.VN,3*Num.Node,1);\nmeasure = [Mea.PN(MeaIdx.PN); Mea.QN(MeaIdx.QN);Mea.VN(MeaIdx.VN)];\nmeasure = measure(:,1);\n\nWPN = SensorError.PN*ones(size(MeaIdx.PN));\nWQN = SensorError.QN*ones(size(MeaIdx.QN));\nWVN = SensorError.VN*ones(size(MeaIdx.VN));\n\nWeight =diag([WPN.^2;WQN.^2;WVN.^2]);\n\nVe1 = reshape(puTrue.Ve,3*Num.Node,1);\nVf1 = reshape(puTrue.Vf,3*Num.Node,1);\nVV1 = [Ve1,Vf1];\nStateVar= reshape(VV1',Num.StateVar * Num.Node,1);\n       \nVe_temp = zeros(Num.Node,3);\nVf_temp = zeros(Num.Node,3);\n\nfor i=1:Num.Node\n    for d=1:3\n        if puTrue.Ve(i,d) == 0\n            Ve_temp(i,d)=0;Vf_temp(i,d)=0;\n        else\n            if d==1\n                Ve_temp(i,d)=0.989*cos(-33.49*pi/180);\n                Vf_temp(i,d)=-0.989*sin(-33.49*pi/180);\n            end\n            if d==2\n                Ve_temp(i,d)=0.993*cos(-153.64*pi/180);\n                Vf_temp(i,d)=-0.993*sin(-153.64*pi/180);\n            end\n            if d==3\n                Ve_temp(i,d)=0.99*cos(86.14*pi/180);\n                Vf_temp(i,d)=-0.99*sin(86.14*pi/180);            \n            end\n        end\n    end\nend\n\nVe1p = reshape(Ve_temp,3*Num.Node,1);\nVf1p = reshape(Vf_temp,3*Num.Node,1);\nVV1p = [Ve1p,-Vf1p];\nInitialValue = reshape(VV1p',Num.StateVar*Num.Node,1);\n\n\nfor i = 1:iterMax\n  % Jocobian matrix\n  [joc_pn,joc_qn] = pnjoc(Num,StateVar,MeaPha,B,G);\n  joc_vn          = vnjoc(Num,StateVar,MeaPha);\n  H = [joc_pn;joc_qn;joc_vn];\n  H(:,2*SlackBus:2*Num.Node:end)=0;   \n  H(:,2*SlackBus-1:2*Num.Node:end)=0; \nindex=i;\n  % MeaEqu\n  [equ_pn,equ_qn] = pnequ(Num,StateVar,MeaPha,B,G);\n  equ_vn = vnequ(Num,StateVar,MeaPha);\n  MeaEqu = [equ_pn;equ_qn;equ_vn];\n  \n  delta_z = measure-MeaEqu;\n  G2 = H'/Weight*delta_z;\n  G3 = H'/Weight*H;    \n  Ginv = pinv(G3);\n  \n  [joc_c,joc_d] = cjoc(Num,B,G,Loc);\n  C = [joc_c;joc_d];\n  C(:,2*SlackBus:2*Num.Node:end)=0;\n  C(:,2*SlackBus-1:2*Num.Node:end)=0;\n  [equ_c,equ_d] = cequ(Num,StateVar,B,G,Loc);\n  delta_c = [-equ_c;-equ_d];  \n  C_temp1 = C*Ginv*C';\n  C_temp2 = pinv(C_temp1);\n  deltaX = Ginv * G2 -Ginv*C'*(C_temp2*(C*Ginv*G2-delta_c)); \n\n  deltaX(abs(deltaX)<1e-8)=0;\n  tol_temp = max(abs(deltaX));\n  if tol_temp < tol\n      break;\n  end\n  StateVar = StateVar + deltaX;\nend\n\ntempVe=StateVar(1:2:6*Num.Node-1);\ntempVf=StateVar(2:2:6*Num.Node);\nseResult.Ve=reshape(tempVe,Num.Node,3);\nseResult.Vf=reshape(tempVf,Num.Node,3);\nseResult.VOL=seResult.Ve+1i*seResult.Vf;\nseResult.AN=angle(seResult.VOL);\nseResult.VN=abs(seResult.VOL);"("V_node"=w14, "P_node"=w13, "I_node"=w12, "NumN"=w10, "NumL"=w9, "Ybus"=w7, "Topology"=w6) -> ("??"=→"error out":errorcluster, "seResult"=→"seResult":T3, "Loc"=→"Loc":cluster{"Zeroinj":i32[][], "Line":dbl[][]}, "Num"=→"Num":T2, "puTrue"=→"puTrue":T1, "index"=→"index":i32)  [unwired: 1 in, 66 out]
    }
  }
